vi "Global_Noise.vi"() -> ()   [LabVIEW 2018]
panel:
  out "Noise":dbl[](graph)
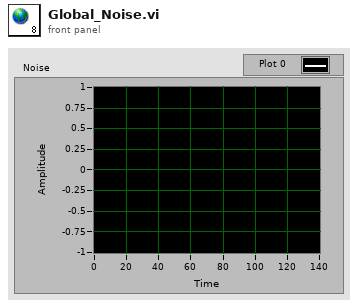
[diagram p1: front panel]
diagram:
